vi "CoboltLaser_AmodEnSet.vi"(6 "Mode":T1, 8 "ErrorIn":errorcluster, 9 "Enabled":bool=TRUE, 10 "CheckResponse":bool=TRUE, 11 "ComPort":refnum<visa-resource-name>) -> (0 "ErrorOut":errorcluster, 1 "Enabled":bool, 2 "Response":string, 3 "ComPortOut":refnum<visa-resource-name>, 4 "ResponseOK":bool)   [LabVIEW 2019]
doc: "Use this template to build a VI to use as a subVI."
uses:
  Programmes Labview/LabScanV1A/DevicesClass/InstrumentsClass/CoboltMLD/CoboltModes.ctl
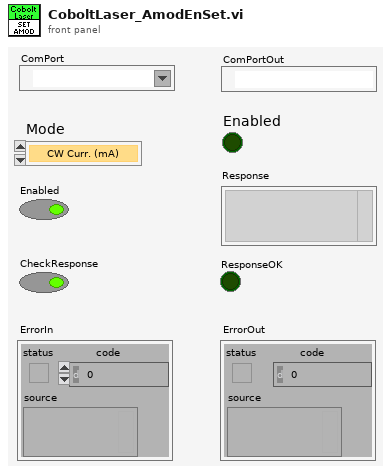
[diagram p1: front panel]
types:
  T1 = typedef "CoboltModes.ctl" = enum16{"CW Curr. (mA)", "CW Pow. (mW)", "Curr. Mod. (mA)", "Pow. Mod. (mW)"}
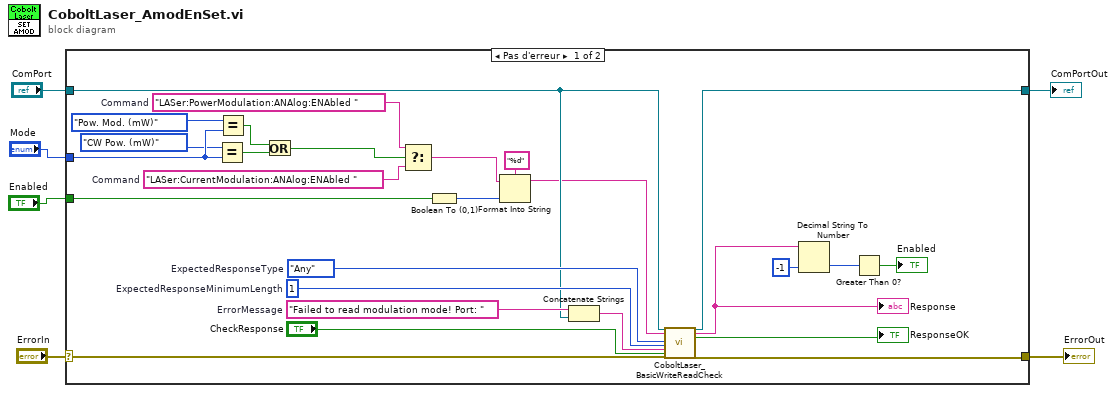
[diagram p0: block diagram]
diagram:
  n1 = case shown="Pas d'erreur" "ErrorIn" {
    selector: "ErrorIn" -> [w33 w35]
    tunnel: [w32 w35] -> w5
    tunnel: "ComPort" -> [w25 w34]
    tunnel: [w24 w34] -> w3
    tunnel: "Enabled" -> [w18 _]
    tunnel: "Mode" -> [w10 _]
    frame No Error {
      w14 = "LASer:CurrentModulation:ANAlog:ENAbled "  # Command
      w30 = 1  # ExpectedResponseMinimumLength
      w31 = enum16{"Any", "Digits Only", "Non-Digits Only"}."Any"  # ExpectedResponseType
      w27 = "Failed to read modulation mode! Port: "  # ErrorMessage
      w15 = "LASer:PowerModulation:ANAlog:ENAbled "  # Command
      n2 = Equal?(x=CoboltModes."CW Pow. (mW)", y=w10) -> (x = y?=w12:bool)
      n3 = Equal?(x=CoboltModes."Pow. Mod. (mW)", y=w10) -> (x = y?=w11:bool)
      n4 = Or(x=w11, y=w12) -> (x .or. y?=w7:bool)
      n5 = Select(t=w15, s=w7, f=w14) -> (s? t:f=w13:string)
      n6 = Boolean To (0,1)(Boolean=w18) -> (0, 1=w17:i16)
      n7 = Format Into String(format string="%d" ("chaîne de format"), initial string=w13, w17) -> (resulting string=w16:string)  [unwired: 1 in, 1 out]
      n8 = Concatenate Strings(w27, w25) -> (w26:string)
      n9 = call <userlib>:"CoboltLaser_BasicWriteReadCheck.vi"("ComPort"=w25, "Command"=w16, "ExpectedResponseType"=w31, "ExpectedResponseMinimumLength"=w30, "ErrorMessage"=w26, "GenerateError"="CheckResponse", "error in (no error)"=w33) -> ("ComPortOut"=w24:refnum<visa-resource-name>, "Response"=w23:string, "ResponseOK"=→"ResponseOK":bool, "error out"=w32:errorcluster)  [unwired: 17 in]
      "Response" <- w23
      n10 = Decimal String To Number(string=w23, default (0L)=-1 ("valeur par défaut (0 I32)")) -> (number=w21:i32)  [unwired: 1 in, 1 out]
      n11 = Greater Than 0?(x=w21) -> (x > 0?=→"Enabled":bool)
    }
    frame Error {
    }
  }
  "ErrorOut" <- w5
  "ComPortOut" <- w3
